vi "Write.vi"(8 "error in (no error)":errorcluster, 10 "PV":refnum<class "PV.lvclass">, 11 "PVConnection in":refnum<class "PVConnection.lvclass">) -> (0 "error out":errorcluster, 3 "PVConnection out":refnum<class "PVConnection.lvclass">)   [LabVIEW 2015, in "CS++ProcessVariables.lvlib" / "PVConnection.lvclass"]
doc: "Publish a process variable."
uses:
  PVConnection.lvclass
  ProcessVariable/PV.lvclass
  PVConnection.lvclass/PVConnection.ctl
  ProcessVariable/PV.lvclass/PV.ctl
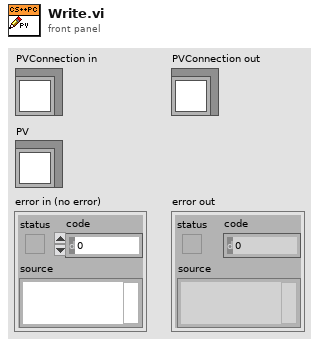
[diagram p1: front panel]
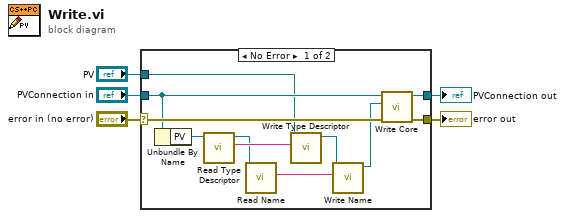
[diagram p0: block diagram]
diagram:
  n1 = case shown="No Error" "error in (no error)" {
    selector: "error in (no error)" -> [w15 w18]
    tunnel: [w14 w18] -> w4
    tunnel: [w16 w17] -> w2
    tunnel: "PVConnection in" -> [w13 w17]
    tunnel: "PV" -> [w11 _]
    frame No Error {
      n2 = Unbundle By Name(w13) -> ("PV"=w12:refnum<class "PV.lvclass">)
      n3 = call "Read Type Descriptor.vi"("PV in"=w12) -> ("Type Descriptor"=w10:string, "PV out"=w9:refnum<class "PV.lvclass">)  [unwired: 8 in, 1 out]
      n4 = call "Read Name.vi"("PV in"=w9) -> ("Name"=w8:string)  [unwired: 8 in, 2 out]
      n5 = call "Write Type Descriptor.vi"("Type Descriptor"=w10, "PV in"=w11) -> ("PV out"=w7:refnum<class "PV.lvclass">)  [unwired: 8 in, 1 out]
      n6 = call "Write Name.vi"("Name"=w8, "PV in"=w7) -> ("PV out"=w6:refnum<class "PV.lvclass">)  [unwired: 8 in, 1 out]
      n7 = call-dynamic "Write Core.vi"("error in (no error)"=w15, "PV"=w6, "PVConnection in"=w13) -> ("error out"=w14:errorcluster, "PVConnection out"=w16:refnum<class "PVConnection.lvclass">)  [unwired: 7 in]
    }
    frame Error {
    }
  }
  "error out" <- w4
  "PVConnection out" <- w2
